vi "Build Tree.vi"(8 "error in":errorcluster, 10 "Tree Refnum":refnum<vi>, 11 "Configuration in":refnum<class "Configuration.lvclass">) -> (0 "error out":errorcluster, 3 "Configuration out":refnum<class "Configuration.lvclass">)   [LabVIEW 2019, in "Configuration.lvlib" / "Configuration.lvclass"]
uses:
  Configuration.lvclass
  Configuration.lvclass/Configuration.ctl
  Accessors/Read Instruments.vi
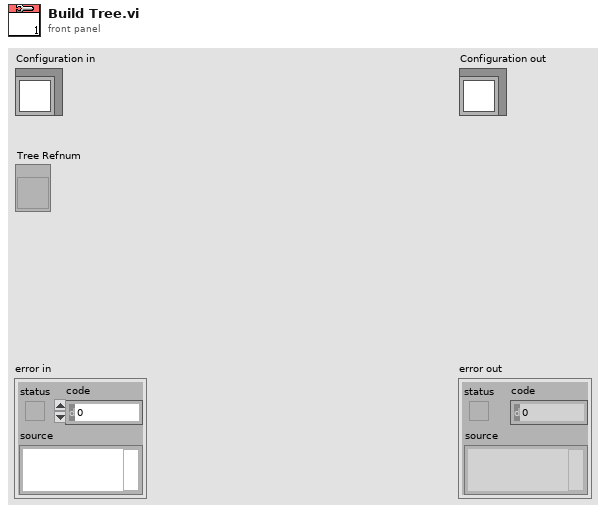
[diagram p1: front panel]
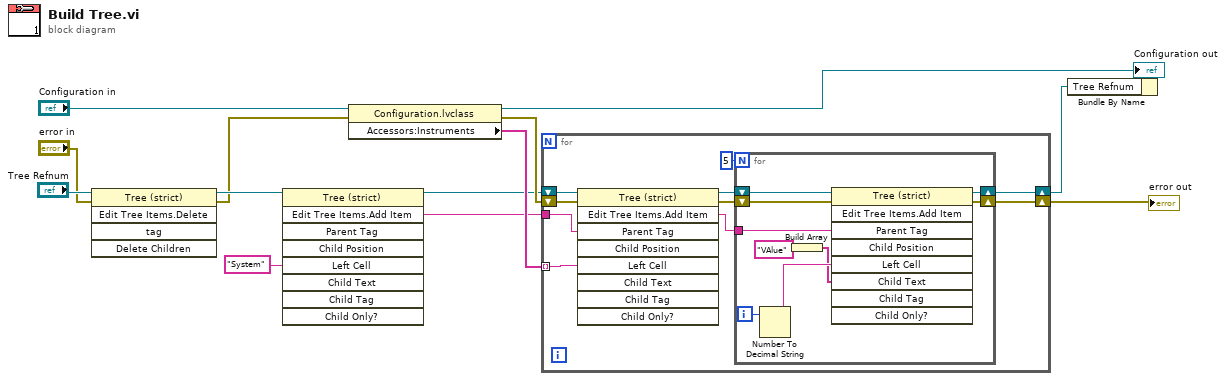
[diagram p0: block diagram]
diagram:
  n1 = invoke class="Tree (strict)" method="Edit Tree Items.Delete"(reference="Tree Refnum", error in="error in") -> (reference out=w10:refnum<vi>, error out=w9:errorcluster)  [unwired: 3 in, 3 out]
  n2 = invoke class="Tree (strict)" method="Edit Tree Items.Add Item"(reference=w10, "Left Cell"="System" ("Parent Tag")) -> (reference out=w7:refnum<vi>, "Edit Tree Items:Add Item"=w5:string)  [unwired: 7 in, 7 out]
  n3 = property class="Configuration.lvclass"(reference="Configuration in", error in=w9) -> (reference out=w12:refnum<class "Configuration.lvclass">, error out=w8:errorcluster, "Accessors:Instruments"=w11:string[])
  n4 = for {
    shift-right: [w19] -> w1
    shift-left: w7 -> [w24]
    tunnel: w11 -> [w21] mode=indexing
    shift-right: [w17] -> w3
    shift-left: w8 -> [w22]
    tunnel: w5 -> [w20]
    n5 = invoke class="Tree (strict)" method="Edit Tree Items.Add Item"(reference=w24, error in=w22, "Parent Tag"=w20, "Left Cell"=w21) -> (reference out=w23:refnum<vi>, error out=w18:errorcluster, "Edit Tree Items:Add Item"=w16:string)  [unwired: 5 in, 6 out]
    n6 = for {
      N: 5 -> [_]
      shift-right: [w32] -> w19
      shift-left: w23 -> [w33]
      shift-right: [w30] -> w17
      shift-left: w18 -> [w31]
      tunnel: w16 -> [w29]
      i -> [w28]
      n7 = Number To Decimal String(number=w28) -> (decimal integer string=w27:string)  [unwired: 1 in]
      n8 = Build Array("VAlue") -> (w25:string[])
      n9 = invoke class="Tree (strict)" method="Edit Tree Items.Add Item"(reference=w33, error in=w31, "Parent Tag"=w29, "Left Cell"=w27, "Child Text"=w25) -> (reference out=w32:refnum<vi>, error out=w30:errorcluster)  [unwired: 4 in, 7 out]
    }
  }
  "error out" <- w3
  n10 = Bundle By Name(cluster=w12, "Tree Refnum"=w1) -> (→"Configuration out":refnum<class "Configuration.lvclass">)
